vi "Global.vi"() -> ()   [LabVIEW 2020]
uses:
  Driver/E5071C/E5071C/E5071C.lvclass
  Driver/PEU/PEU/PEU.lvclass
panel:
  in  "Freqs":dbl[](array[numeric])
  in  "BasePath":path
  in  "Sub Panel":refnum<vi>
  in  "PEU":refnum<class "PEU.lvclass">
  in  "E5071C":refnum<class "E5071C.lvclass">
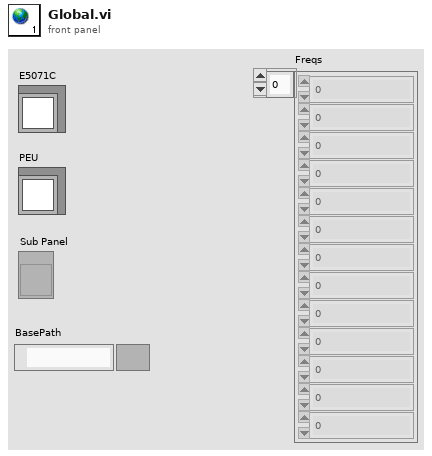
[diagram p1: front panel]
diagram:
